vi "Process.vi"(8 "error in (no error)":errorcluster, 11 "SMO.UI":refnum<class "SMO.UI.Template.lvclass">) -> (0 "error out":errorcluster, 3 "SMO.UI out":refnum<class "SMO.UI.Template.lvclass">)   [LabVIEW 2013, in "SMO.UI.Template.lvclass"]
uses:
  SMO.UI.Template.lvclass
  SMO/Typedefs/Parent Call--Enum.ctl
  SMO.UI/SMO.UI.lvclass
  SMO/SMO.lvclass
panel:
  in  "OK":bool
  # "UI Template"
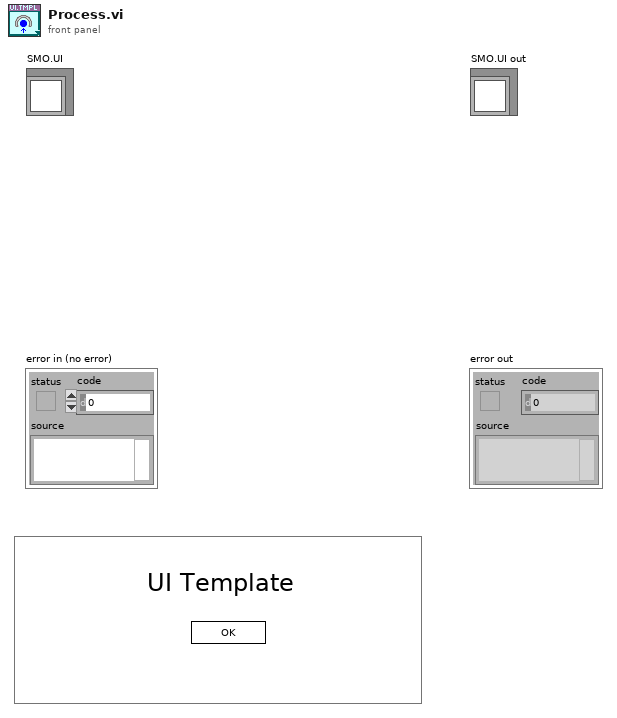
[diagram p1: front panel]
types:
  T1 = typedef "SMO.lvclass/Parent Call--Enum.ctl" = enum16{"Allows parent to run", "Does not request parent to run"}
  T2 = enum32{"invalid app kind", "Development System", "Run Time System", "Student Edition", "Embedded LabVIEW", "Evaluation", "Custom"}
  T3 = enum32{"Invalid", "Standard", "Closed", "Hidden", "Minimized", "Maximized"}
  T4 = cluster{"Core":cluster{"Current VI Reference":refnum<vi>, "Close Panel on Exit?":bool, "error":errorcluster}, "Self Ref":refnum<class "SMO.UI.Template.lvclass">}
  T5 = cluster{"Current VI Reference":refnum<vi>, "Close Panel on Exit?":bool, "error":errorcluster}
  T6 = typedef "SMO.lvclass/Protected Events.ctl" = cluster{"StopProcesses":refnum<user-event>, "AbortProcesses":refnum<user-event>}
  T7 = cluster{"Event Registration Refnum":refnum<event-registration>, "SMO.UI Public Events":refnum<event-registration>}
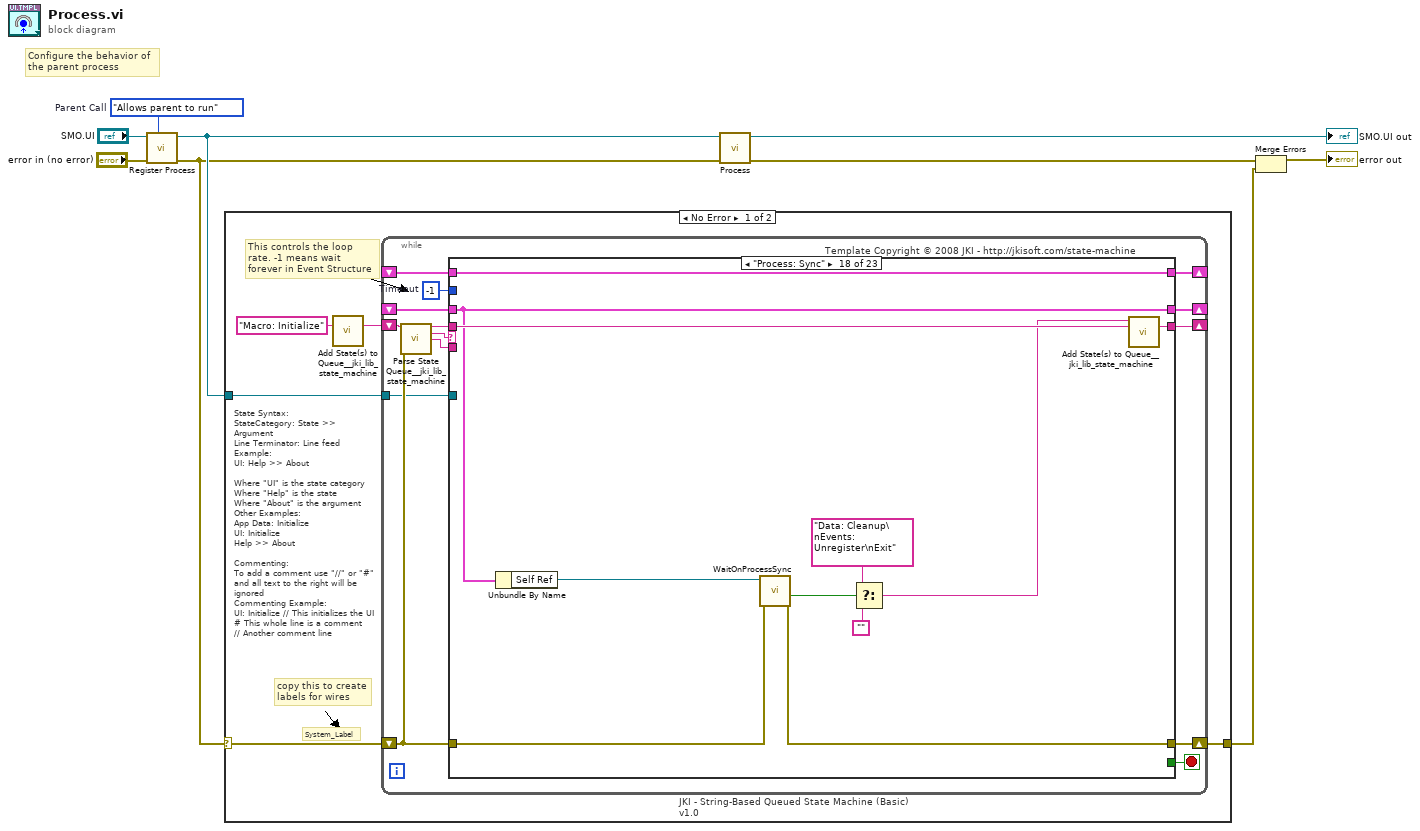
[diagram p0: block diagram]
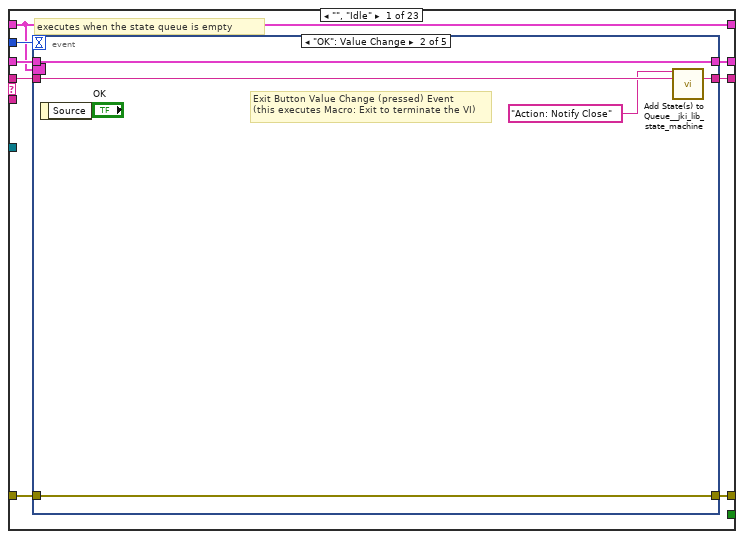
[diagram p2: hidden frame]
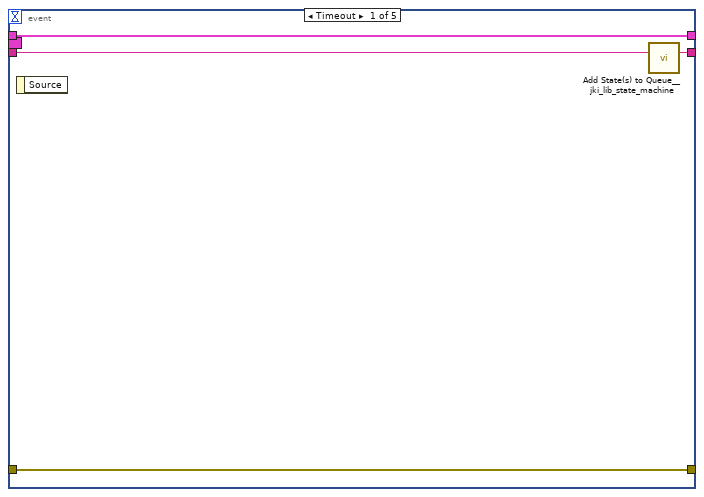
[diagram p3: hidden frame]
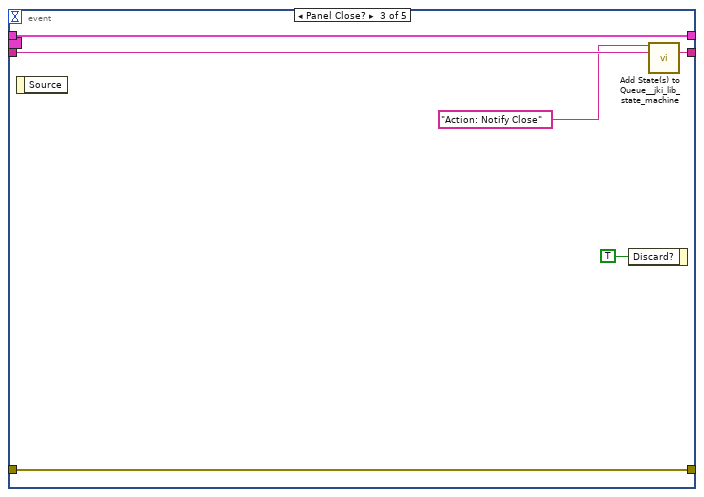
[diagram p4: hidden frame]
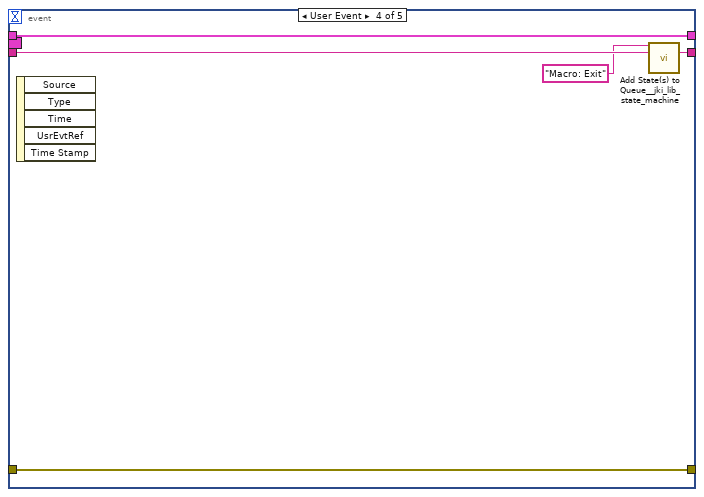
[diagram p5: hidden frame]
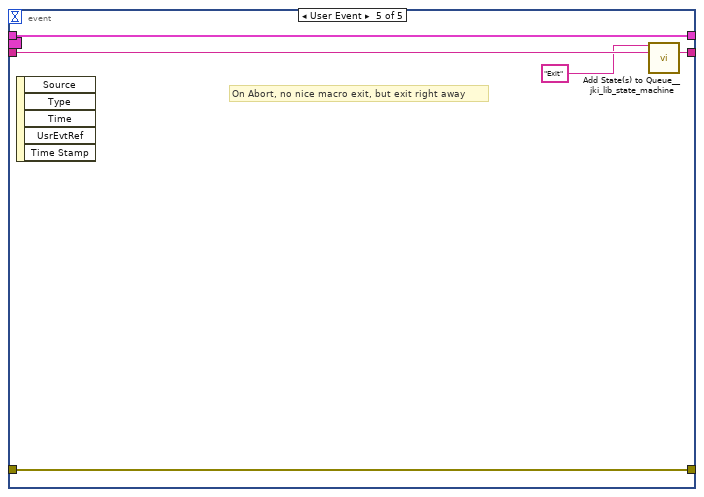
[diagram p6: hidden frame]
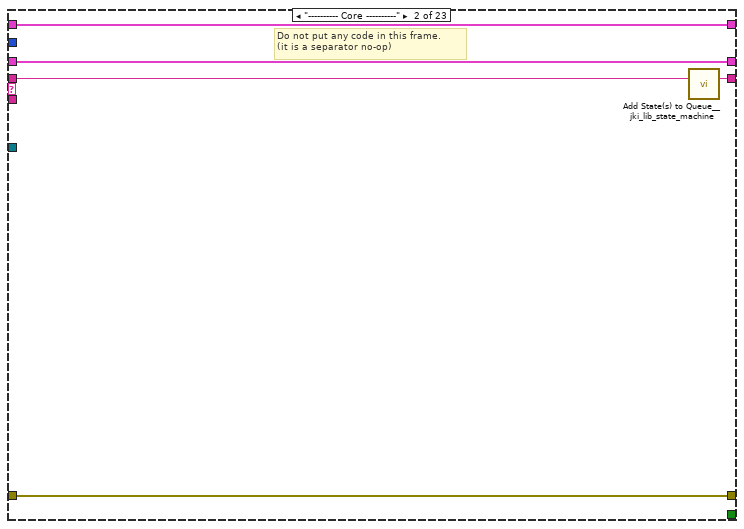
[diagram p7: hidden frame]
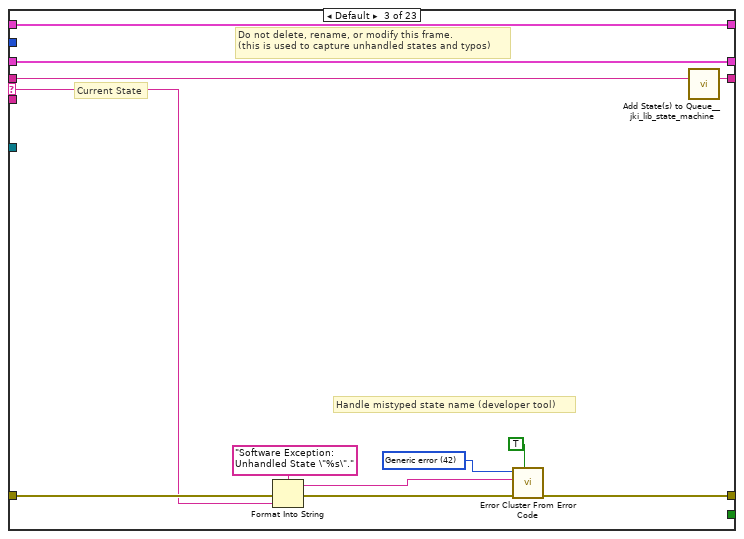
[diagram p8: hidden frame]
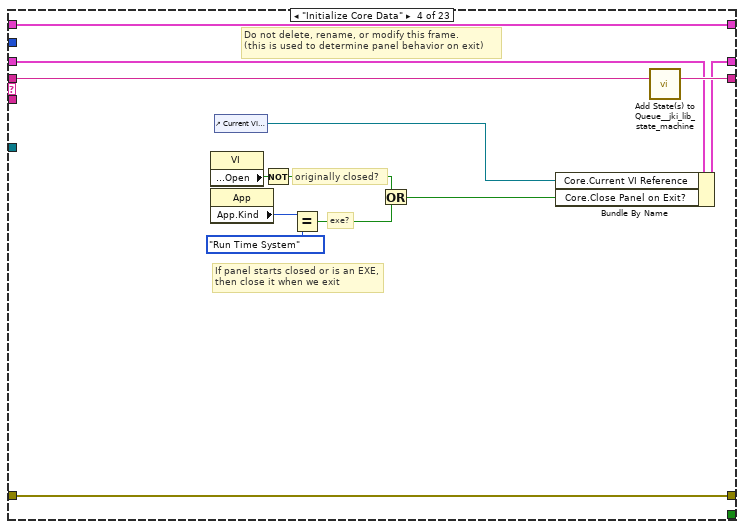
[diagram p9: hidden frame]
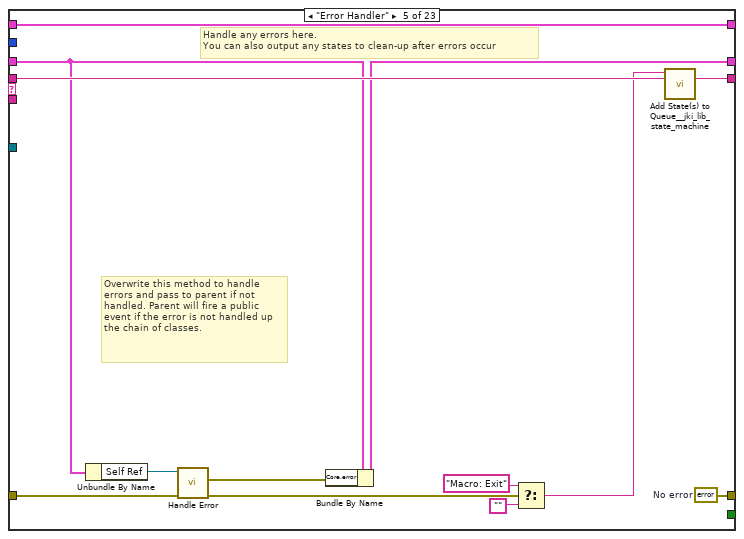
[diagram p10: hidden frame]
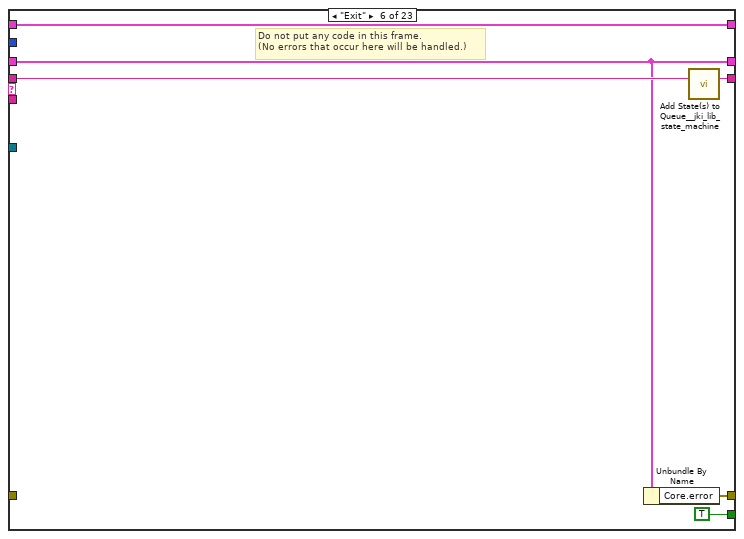
[diagram p11: hidden frame]
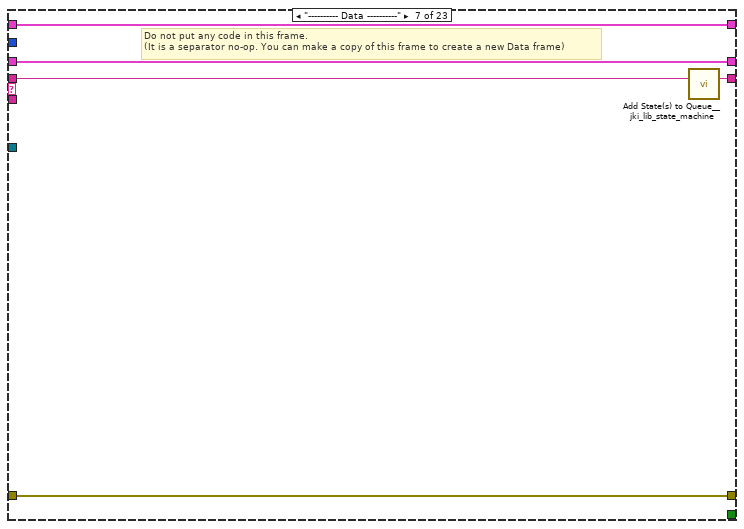
[diagram p12: hidden frame]
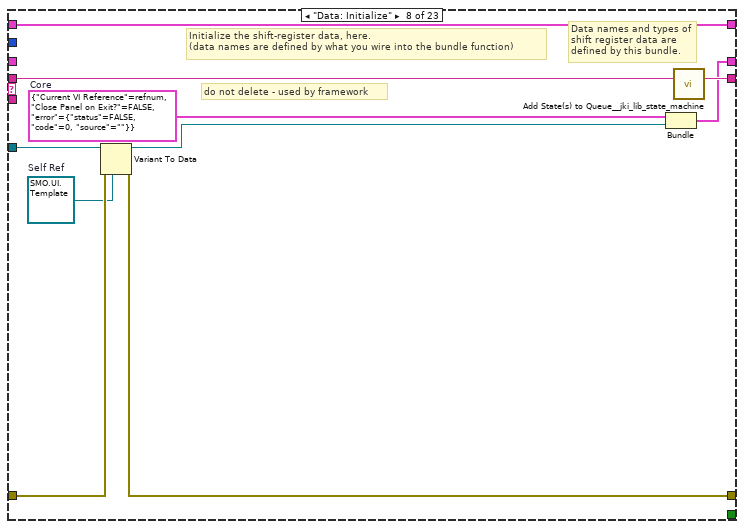
[diagram p13: hidden frame]
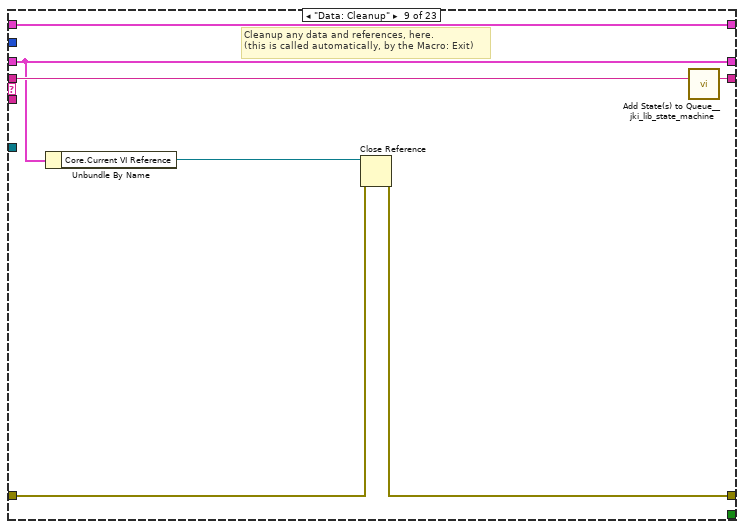
[diagram p14: hidden frame]
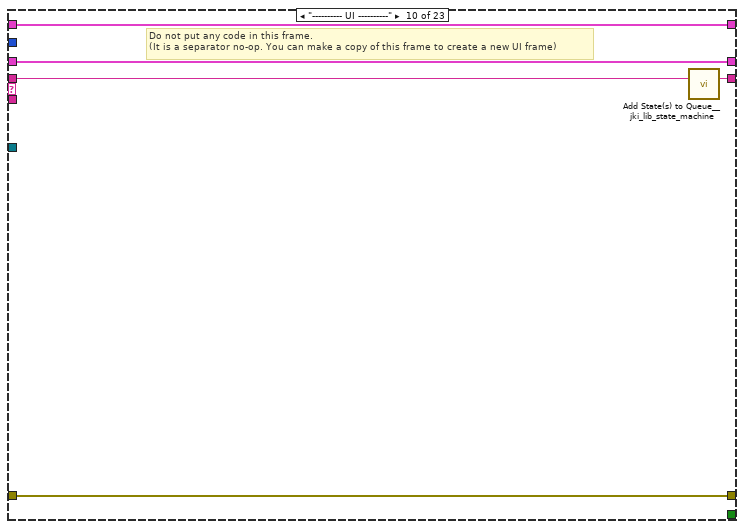
[diagram p15: hidden frame]
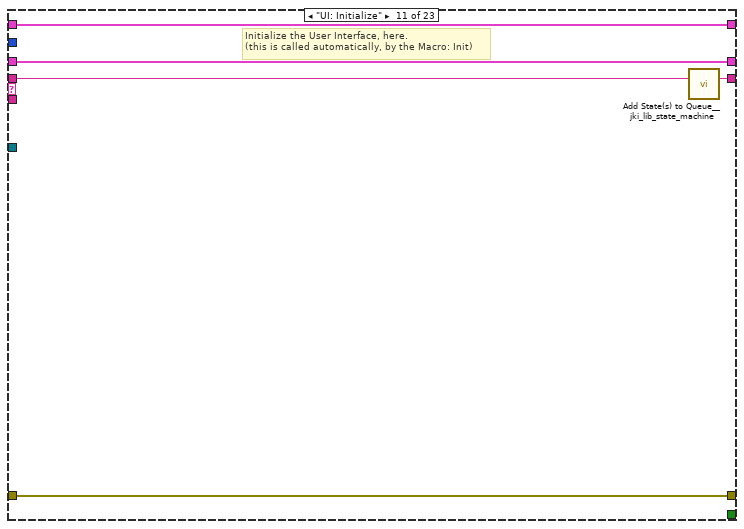
[diagram p16: hidden frame]
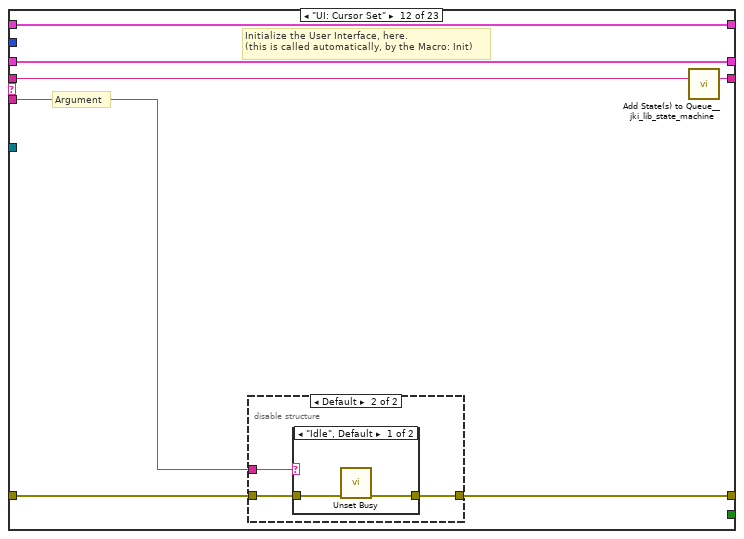
[diagram p17: hidden frame]
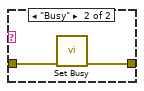
[diagram p19: hidden frame]
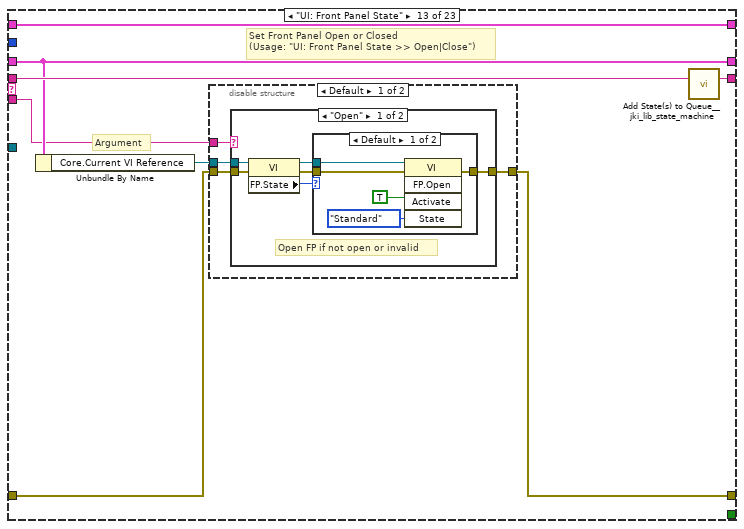
[diagram p20: hidden frame]
diagram:
  w1 = Parent_Call--Enum."Allows parent to run"  # Parent Call
  # "Configure the behavior of the parent process"
  n1 = call "Register Process.vi"("Parent Call"=w1, "error in (no error)"="error in (no error)", "SMO"="SMO.UI") -> ("error out"=w3:errorcluster, "SMO out"=w4:refnum<class "SMO.UI.Template.lvclass">)  [unwired: 7 in]
  n2 = case shown="No Error" w3 {
    selector: w3 -> [w11 w271]
    tunnel: w4 -> [w12 _]
    tunnel: [w10 w271] -> w2
    frame No Error {
      # "State Syntax:\nStateCategory: State >> Argument\nLine Terminator: Line feed\nExample:\nUI: Help >> About\n\nWhere \"UI\" is the state category\nWhere \"Help\" is the state\nWhere \"About\" is the argument\nOther Examples:\nApp Data: Initialize\nUI: Initialize\nHelp >> About\n\nCommenting:\nTo add a comment use \"//\" or \"#\" and all text to the right will be ignored\nCommenting Example:\nUI: Initialize // This initializes the UI\n# This whole line is a comment\n// Another comment line"
      # "copy this to create labels for wires"
      # "This controls the loop rate. -1 means wait forever in Event Structure"
      # "System_Label"
      n3 = call <vilib>:"Add State(s) to Queue__jki_lib_state_machine.vi"("State(s) in (\"\")"="Macro: Initialize") -> ("States Out"=w14:string)  [unwired: 14 in]
      n4 = while "JKI - String-Based Queued State Machine (Basic) v1.0" {
        shift-right: [w21] -> _
        shift-left: _ -> [w20]
        shift-right: [w24] -> w10
        shift-left: w11 -> [w18]
        shift-right: [w23] -> _
        shift-left: w14 -> [w25]
        tunnel: w12 -> [w17]
        shift-right: [w16] -> _
        shift-left: _ -> [w15]
        stop <- w22 stop-if-true
        w19 = -1  # Timeout
        # "Template Copyright © 2008 JKI - http://jkisoft.com/state-machine"
        n5 = call <vilib>:"Parse State Queue__jki_lib_state_machine.vi"("State Queue"=w25, "Error In (no error)"=w18) -> ("Remaining States"=w27:string, "Current State"=w28:string, "Arguments"=w26:string)  [unwired: 11 in]
        n6 = case shown="\"Process: Sync\"" w28 {
          selector: w28 -> [_ _ w68 _ _ _ _ _ _ _ _ _ _ _ _ _ _ _ _ _ _ _ _]
          tunnel: w27 -> [w36 w66 w72 w91 w104 w110 w115 w125 w132 w137 w142 w149 w165 w197 w206 w217 w222 w233 w238 w252 w258 w263 w270]
          tunnel: w26 -> [_ _ _ _ _ _ _ _ _ _ _ w143 w158 _ _ _ _ _ _ _ _ _ _]
          tunnel: w20 -> [w34 w63 w70 w82 w95 w106 w112 _ w127 w134 w140 w147 w163 w194 w202 w208 w219 w229 w235 w250 w256 w260 w266]
          tunnel: [w33 w64 w74 w88 w92 w105 w113 w116 w128 w135 w139 w144 w160 w195 w204 w215 w220 w230 w236 w239 w254 w261 w264] -> w24
          tunnel: w18 -> [w32 w64 w73 w88 w96 _ w113 w122 w129 w135 w139 w145 w161 w195 w204 w215 w220 w227 w236 w243 w254 w261 w265]
          tunnel: [w35 w65 w71 w90 w103 w109 w114 w124 w131 w136 w141 w148 w164 w196 w205 w216 w221 w232 w237 w251 w257 w262 w269] -> w23
          tunnel: [_ _ _ _ _ TRUE _ _ _ _ _ _ _ _ _ _ _ _ _ _ _ _ _] -> w22
          tunnel: [w31 w63 w70 w89 w94 w106 w112 w123 w127 w134 w140 w147 w163 w194 w202 w208 w219 w229 w235 w250 w256 w260 w266] -> w21
          tunnel: w19 -> [w30 _ _ _ _ _ _ _ _ _ _ _ _ _ _ _ _ _ _ _ _ _ _]
          tunnel: w17 -> [_ _ _ _ _ _ _ w121 _ _ _ _ _ _ _ _ _ _ _ _ _ _ _]
          tunnel: [w29 w62 w67 w79 w102 w107 w111 w120 w126 w133 w138 w146 w162 w193 w203 w209 w218 w231 w234 w246 w255 w259 w268] -> w16
          tunnel: w15 -> [w29 w62 w67 w79 w102 w107 w111 w120 w126 w133 w138 w146 w162 w193 w203 w209 w218 w231 w234 _ w255 w259 w268]
          frame "", "Idle" {
            # "executes when the state queue is empty"
            n7 = event shown="[1] \"OK\": Value Change" {
              selector: w29 -> [_ _ _ _ _]
              dyn-events: _ -> [_ _ _ _ _]
              timeout: w30 -> [_ _ _ _ _]
              tunnel: w36 -> [w40 w45 w51 w56 w61]
              tunnel: [w39 w44 w50 w55 w60] -> w35
              tunnel: w34 -> [w37 w42 w48 w53 w58]
              tunnel: [w38 w43 w47 w54 w59] -> w33
              tunnel: w32 -> [w38 w43 w47 w54 w59]
              tunnel: [w37 w42 w48 w53 w58] -> w31
              event Timeout {
                n8 = event-data() -> ()  [unwired: 1 in, 1 out]
                n9 = call <vilib>:"Add State(s) to Queue__jki_lib_state_machine.vi"("State(s) in (\"\")"=w40) -> ("States Out"=w39:string)  [unwired: 14 in]
              }
              event "OK": Value Change {
                # "Exit Button Value Change (pressed) Event\n(this executes Macro: Exit to terminate the VI)"
                n10 = event-data() -> ()  [unwired: 1 in, 1 out]
                n11 = call <vilib>:"Add State(s) to Queue__jki_lib_state_machine.vi"("State(s) in Front (\"\")"="Action: Notify Close", "State(s) in (\"\")"=w45) -> ("States Out"=w44:string)  [unwired: 13 in]
              }
              event Panel Close? {
                n12 = event-data() -> ()  [unwired: 1 in, 1 out]
                n13 = event-data("Discard?"=TRUE) -> ()  [unwired: 1 in, 1 out]
                n14 = call <vilib>:"Add State(s) to Queue__jki_lib_state_machine.vi"("State(s) in Front (\"\")"="Action: Notify Close" ("State(s) in Front (\"\")"), "State(s) in (\"\")"=w51) -> ("States Out"=w50:string)  [unwired: 13 in]
              }
              event User Event {
                n15 = event-data() -> ()  [unwired: 1 in, 5 out]
                n16 = call <vilib>:"Add State(s) to Queue__jki_lib_state_machine.vi"("State(s) in Front (\"\")"="Macro: Exit", "State(s) in (\"\")"=w56) -> ("States Out"=w55:string)  [unwired: 13 in]
              }
              event User Event {
                # "On Abort, no nice macro exit, but exit right away"
                n17 = event-data() -> ()  [unwired: 1 in, 5 out]
                n18 = call <vilib>:"Add State(s) to Queue__jki_lib_state_machine.vi"("State(s) in Front (\"\")"="Exit", "State(s) in (\"\")"=w61) -> ("States Out"=w60:string)  [unwired: 13 in]
              }
            }
          }
          frame "---------- Core ----------" {
            # "Do not put any code in this frame.\n(it is a separator no-op)"
            n19 = call <vilib>:"Add State(s) to Queue__jki_lib_state_machine.vi"("State(s) in (\"\")"=w66) -> ("States Out"=w65:string)  [unwired: 14 in]
          }
          frame Default {
            w77 = 42 items=["No error", "Argument error", "Memory is full", "Out of zone", "End of file", "File already open", "Generic file I/O error", "File not found", "File permission error", "Disk is full", "Duplicate path", "Too many files open", "System feature not enabled", "Resource file not found", "Cannot add resource", "Resource not found", "Image not found", "Image memory error", "Pen does not exist", "Config type invalid", "Config token not found", "Config parse error", "Config memory error", "Bad external code format", "Bad external code offset", "External code not present", "Null window", "Destroy window error", "Null menu", "Print aborted", "Bad print record", "Print driver error", "Windows error during printing", "Memory error during printing", "Print dialog error", "Generic print error", "Invalid device refnum", "Device not found", "Device parameter error", "Device unit error", "Cannot open device", "Device call aborted", "Generic error", "Cancelled by user", "Object ID too low", "Object ID too high", "Object not in heap", "Unknown heap", "Unknown object (invalid DefProc)", "Unknown object (DefProc not in table)", "Message out of range", "Invalid (null) method", "Unknown message", "Manager call not supported", "Bad address", "Network operation in progress", "Network operation timed out", "Connection is busy", "Network attribute not supported", "Network error", "Address in use", "System out of memory", "Connection aborted", "Connection refused", "Not connected", "Already connected", "Connection closed", "Initialization error (interapplication manager)", "Bad occurrence", "Wait on unbound occurrence handler", "Occurrence queue overflow", "Datalog type conflict", "Unused", "Unrecognized type (interapplication manager)", "Memory corrupt", "Failed to make temporary DLL", "Old CIN version", "Drag socket not found", "Failed to load drop-object", "Failed to register OLE object", "Failed to release OLE object", "Format specifier type mismatch", "Unknown format specifier", "Too few format specifiers", "Too many format specifiers", "Scan failed", "Newer CIN version", "Error converting to variant", "Runtime menu error", "Password tampered", "Variant attribute not found", "Incompatible variant data type", "Event data is not available", "Event Store is not present", "Occurrence is not found", "Event Queue is not created", "Event info is not available", "Refnum passed is NULL", "Error retrieving Class GUID", "Error retrieving CoClass GUID", "Error retrieving TypeLib GUID.", "Bad built application magic bytes.", "Specific driver is different from the specific driver associated with the Logical Name.", "There is no session opened to the class driver.", "Max Error", "MAX - Error with config objects", "MAX - Error loading configuration", "MAX - Group not supported"]
            # "Current State"
            # "Do not delete, rename, or modify this frame.\n(this is used to capture unhandled states and typos)"
            # "Handle mistyped state name (developer tool)"
            n20 = Format Into String(format string="Software Exception: Unhandled State \"%s\"." ("message"), error in=w73, w68) -> (resulting string=w76:string, error out=w75:errorcluster)  [unwired: 1 in]
            n21 = call <vilib>:"Error Cluster From Error Code.vi"("show call chain? (False)"=TRUE, "error in (no error)"=w75, "error message (\"\")"=w76, "error code (0)"=w77) -> ("error out"=w74:errorcluster)  [unwired: 5 in]
            n22 = call <vilib>:"Add State(s) to Queue__jki_lib_state_machine.vi"("State(s) in (\"\")"=w72) -> ("States Out"=w71:string)  [unwired: 14 in]
          }
          frame "Initialize Core Data" {
            # "Do not delete, rename, or modify this frame.\n(this is used to determine panel behavior on exit)"
            # "originally closed?"
            # "exe?"
            # "If panel starts closed or is an EXE, then close it when we exit"
            n23 = property class="VI"() -> ("Front Panel.Open"=w87:bool)  [unwired: 2 in, 2 out]
            n24 = property class="App"() -> ("App.Kind"=w86:T2)  [unwired: 2 in, 2 out]
            n25 = control-ref of="Current VI Reference"() -> (w80:refnum<vi>)
            n26 = Not(x=w87) -> (.not. x?=w84:bool)
            n27 = Equal?(x=w86, y=T2."Run Time System" ("Application:Kind")) -> (x = y?=w83:bool)
            n28 = Or(x=w84, y=w83) -> (x .or. y?=w81:bool)
            n29 = Bundle By Name(cluster=w82, "Core.Current VI Reference"=w80, "Core.Close Panel on Exit?"=w81) -> (w89:T4)
            n30 = call <vilib>:"Add State(s) to Queue__jki_lib_state_machine.vi"("State(s) in (\"\")"=w91) -> ("States Out"=w90:string)  [unwired: 14 in]
          }
          frame "Error Handler" {
            w92 = errorcluster {"status"=FALSE, "code"=0, "source"=""}  # No error
            # "Overwrite this method to handle errors and pass to parent if not handled. Parent will fire a public event if the error is not handled up the chain of classes."
            # "Handle any errors here.\nYou can also output any states to clean-up after errors occur"
            n31 = Unbundle By Name(w95) -> ("Self Ref"=w97:refnum<class "SMO.UI.Template.lvclass">)
            n32 = call-dynamic "Handle Error.vi"("error in"=w96, "SMO"=w97) -> ("handling error"=w100:errorcluster, "Unhandled error"=w101:errorcluster)  [unwired: 7 in, 1 out]
            n33 = Bundle By Name(cluster=w95, "Core.error"=w101) -> (w94:T4)
            n34 = Select(t="Macro: Exit", s=w100, f="") -> (s? t:f=w93:string)
            n35 = call <vilib>:"Add State(s) to Queue__jki_lib_state_machine.vi"("State(s) in Front (\"\")"=w93, "State(s) in (\"\")"=w104) -> ("States Out"=w103:string)  [unwired: 13 in]
          }
          frame "Exit" {
            # "Do not put any code in this frame.\n(No errors that occur here will be handled.)"
            n36 = Unbundle By Name(w106) -> ("Core.error"=w105:errorcluster)
            n37 = call <vilib>:"Add State(s) to Queue__jki_lib_state_machine.vi"("State(s) in (\"\")"=w110) -> ("States Out"=w109:string)  [unwired: 14 in]
          }
          frame "---------- Data ----------" {
            # "Do not put any code in this frame.\n(It is a separator no-op. You can make a copy of this frame to create a new Data frame)"
            n38 = call <vilib>:"Add State(s) to Queue__jki_lib_state_machine.vi"("State(s) in (\"\")"=w115) -> ("States Out"=w114:string)  [unwired: 14 in]
          }
          frame "Data: Initialize" {
            w117 = T5 {"Current VI Reference"=refnum, "Close Panel on Exit?"=FALSE, "error"={"status"=FALSE, "code"=0, "source"=""}}  # Core
            w119 = refnum<class "SMO.UI.Template.lvclass"> refnum  # Self Ref
            # "do not delete - used by framework"
            # "Data names and types of shift register data are defined by this bundle."
            # "Initialize the shift-register data, here.\n(data names are defined by what you wire into the bundle function)"
            n39 = Variant To Data(error in=w122, type=w119, Variant=w121) -> (data=w118:refnum<class "SMO.UI.Template.lvclass">, error out=w116:errorcluster)
            n40 = Bundle("Core"=w117, "Self Ref"=w118) -> (w123:T4)  [unwired: 1 in]
            n41 = call <vilib>:"Add State(s) to Queue__jki_lib_state_machine.vi"("State(s) in (\"\")"=w125) -> ("States Out"=w124:string)  [unwired: 14 in]
          }
          frame "Data: Cleanup" {
            # "Cleanup any data and references, here.\n(this is called automatically, by the Macro: Exit)"
            n42 = Unbundle By Name(w127) -> ("Core.Current VI Reference"=w130:refnum<vi>)
            n43 = Close Reference(reference=w130, error in (no error)=w129) -> (error out=w128:errorcluster)
            n44 = call <vilib>:"Add State(s) to Queue__jki_lib_state_machine.vi"("State(s) in (\"\")"=w132) -> ("States Out"=w131:string)  [unwired: 14 in]
          }
          frame "---------- UI ----------" {
            # "Do not put any code in this frame.\n(It is a separator no-op. You can make a copy of this frame to create a new UI frame)"
            n45 = call <vilib>:"Add State(s) to Queue__jki_lib_state_machine.vi"("State(s) in (\"\")"=w137) -> ("States Out"=w136:string)  [unwired: 14 in]
          }
          frame "UI: Initialize" {
            # "Initialize the User Interface, here.\n(this is called automatically, by the Macro: Init)"
            n46 = call <vilib>:"Add State(s) to Queue__jki_lib_state_machine.vi"("State(s) in (\"\")"=w142) -> ("States Out"=w141:string)  [unwired: 14 in]
          }
          frame "UI: Cursor Set" {
            # "Argument"
            # "Initialize the User Interface, here.\n(this is called automatically, by the Macro: Init)"
            n47 = disable-structure shown="Default" {
              disable-tunnel: w145 -> [w150 w153]
              disable-tunnel: [w150 w152] -> w144
              disable-tunnel: w143 -> [_ w151]
              frame condition #0 {
              }
              frame condition #1 (active) {
                n48 = case shown="\"Idle\", Default" w151 {
                  tunnel: w153 -> [w155 w157]
                  tunnel: [w154 w156] -> w152
                  frame "Idle", Default {
                    n49 = call <vilib>:"Unset Busy.vi"("error in (no error)"=w155) -> ("error out"=w154:errorcluster)  [unwired: 10 in]
                  }
                  frame "Busy" {
                    n50 = call <vilib>:"Set Busy.vi"("error in (no error)"=w157) -> ("error out"=w156:errorcluster)  [unwired: 9 in, 1 out]
                  }
                }
              }
            }
            n51 = call <vilib>:"Add State(s) to Queue__jki_lib_state_machine.vi"("State(s) in (\"\")"=w149) -> ("States Out"=w148:string)  [unwired: 14 in]
          }
          frame "UI: Front Panel State" {
            # "Argument"
            # "Set Front Panel Open or Closed\n(Usage: \"UI: Front Panel State >> Open|Close\")"
            n52 = Unbundle By Name(w163) -> ("Core.Current VI Reference"=w159:refnum<vi>)
            n53 = disable-structure shown="Default" {
              disable-tunnel: w161 -> [w169 w192]
              disable-tunnel: [w168 w192] -> w160
              disable-tunnel: w159 -> [w167 _]
              disable-tunnel: w158 -> [w166 _]
              frame condition #0 (active) {
                n54 = case shown="\"Open\"" w166 {
                  tunnel: w169 -> [w173 w186]
                  tunnel: [w175 w187] -> w168
                  tunnel: w167 -> [w174 w184]
                  frame "Open" {
                    # "Open FP if not open or invalid"
                    n55 = property class="VI"(reference=w174, error in=w173) -> (reference out=w171:refnum<vi>, error out=w172:errorcluster, "FP.State"=w170:T3)
                    n56 = case shown="Default" w170 {
                      tunnel: [w178 w181] -> w175
                      tunnel: w172 -> [w177 w181]
                      tunnel: w171 -> [w176 _]
                      frame Default {
                        n57 = invoke class="VI" method="FP.Open"(reference=w176, error in=w177, "Activate"=TRUE, "State"=T3."Standard") -> (error out=w178:errorcluster)  [unwired: 1 in, 4 out]
                      }
                      frame "Invalid", "Standard" {
                      }
                    }
                  }
                  frame "Close", Default {
                    # "Close FP is not Closed or Invalid"
                    n58 = property class="VI"(reference=w184, error in=w186) -> (reference out=w183:refnum<vi>, error out=w185:errorcluster, "FP.State"=w182:T3)
                    n59 = case shown="Default" w182 {
                      tunnel: [w188 w191] -> w187
                      tunnel: w185 -> [w188 w190]
                      tunnel: w183 -> [_ w189]
                      frame "Invalid", "Closed" {
                      }
                      frame Default {
                        n60 = invoke class="VI" method="FP.Close"(reference=w189, error in=w190) -> (error out=w191:errorcluster)  [unwired: 1 in, 2 out]
                      }
                    }
                  }
                }
              }
              frame condition #1 {
              }
            }
            n61 = call <vilib>:"Add State(s) to Queue__jki_lib_state_machine.vi"("State(s) in (\"\")"=w165) -> ("States Out"=w164:string)  [unwired: 14 in]
          }
          frame "---------- Macro ----------" {
            # "Do not put any code in this frame.\n(It is a separator no-op. You can make a copy of this frame to create a new Macro frame)"
            n62 = call <vilib>:"Add State(s) to Queue__jki_lib_state_machine.vi"("State(s) in (\"\")"=w197) -> ("States Out"=w196:string)  [unwired: 14 in]
          }
          frame "Macro: Initialize" {
            w200 = "UI: Initialize\n//UI: Front Panel State >> Open"  # UI: Initialize //UI: Front Panel State >> Open
            # "Initialization Macro\n(This is called once, when the VI starts)"
            n63 = call <vilib>:"Add State(s) to Queue__jki_lib_state_machine.vi"("State(s) in Front (\"\")"="Data: Initialize\nInitialize Core Data\nEvents: Register", "State(s) in (\"\")"="Process: Sync", "State(s) at Back (\"\")"=w200) -> ("States Out"=w199:string)  [unwired: 12 in]
            n64 = call <vilib>:"Add State(s) to Queue__jki_lib_state_machine.vi"("State(s) in Front (\"\")"=w199, "State(s) in (\"\")"=w206) -> ("States Out"=w205:string)  [unwired: 13 in]
          }
          frame "Macro: Exit" {
            # "Exit Macro\n(This is called once, when the VI exits)"
            n65 = Unbundle By Name(w208) -> ("Core.Close Panel on Exit?"=w214:bool)
            n66 = Select(t="//UI: Front Panel State >> Close", s=w214, f="") -> (s? t:f=w211:string)
            n67 = call <vilib>:"Add State(s) to Queue__jki_lib_state_machine.vi"("State(s) in (\"\")"=w211, "State(s) at Back (\"\")"="Data: Cleanup\nEvents: Unregister\nProcess: Sync\nExit") -> ("States Out"=w210:string)  [unwired: 13 in]
            n68 = call <vilib>:"Add State(s) to Queue__jki_lib_state_machine.vi"("State(s) in Front (\"\")"=w210, "State(s) in (\"\")"=w217) -> ("States Out"=w216:string)  [unwired: 13 in]
          }
          frame "---------- Process ----------" {
            # "Template Separator\n(You can make a copy of, or modify, this frame)"
            n69 = call <vilib>:"Add State(s) to Queue__jki_lib_state_machine.vi"("State(s) in (\"\")"=w222) -> ("States Out"=w221:string)  [unwired: 14 in]
          }
          frame "Process: Sync" {
            n70 = Unbundle By Name(w229) -> ("Self Ref"=w228:refnum<class "SMO.UI.Template.lvclass">)
            n71 = call "WaitOnProcessSync.vi"("error in (no error)"=w227, "SMO"=w228) -> ("error out"=w230:errorcluster, "Don't run?"=w226:bool)  [unwired: 7 in, 1 out]
            n72 = Select(t="Data: Cleanup\nEvents: Unregister\nExit", s=w226, f="") -> (s? t:f=w223:string)
            n73 = call <vilib>:"Add State(s) to Queue__jki_lib_state_machine.vi"("State(s) in Front (\"\")"=w223, "State(s) in (\"\")"=w233) -> ("States Out"=w232:string)  [unwired: 13 in]
          }
          frame "---------- Events ----------" {
            # "Template Separator\n(You can make a copy of, or modify, this frame)"
            n74 = call <vilib>:"Add State(s) to Queue__jki_lib_state_machine.vi"("State(s) in (\"\")"=w238) -> ("States Out"=w237:string)  [unwired: 14 in]
          }
          frame "Events: Register" {
            # "Base Class Protected Events"
            # "Your code here.\n(You can make a copy of, or modify, this frame)"
            n75 = Unbundle By Name(w250) -> ("Self Ref"=w248:refnum<class "SMO.UI.Template.lvclass">)
            n76 = call "GetProtectedEvents.vi"("SMO"=w248) -> ("error out"=w240:errorcluster, "SMO Protected Events"=w249:T6, "SMO out"=w245:refnum<class "SMO.UI.Template.lvclass">)  [unwired: 8 in]
            n77 = call "SMO.UI.GetPublicEventsRegistration.vi"("SMO.UI"=w245) -> ("error out"=w241:errorcluster, "SMO.UI Public Events"=w244:refnum<event-registration>)  [unwired: 8 in, 1 out]
            n78 = register-events(w249) -> (reference out=w247:refnum<event-registration>, error out=w242:errorcluster)  [unwired: 2 in]
            n79 = Merge Errors(w242, w241, w240, w243) -> (w239:errorcluster)
            n80 = Bundle("Event Registration Refnum"=w247, "SMO.UI Public Events"=w244) -> (w246:T7)  [unwired: 1 in]
            n81 = call <vilib>:"Add State(s) to Queue__jki_lib_state_machine.vi"("State(s) in (\"\")"=w252) -> ("States Out"=w251:string)  [unwired: 14 in]
          }
          frame "Events: Unregister" {
            n82 = Unregister For Events(event registration refnum=w255, error in=w254) -> (error out=w253:errorcluster)
            n83 = call <vilib>:"Clear Errors.vi"("error in (no error)"=w253) -> ()  [unwired: 6 in, 1 out]
            n84 = call <vilib>:"Add State(s) to Queue__jki_lib_state_machine.vi"("State(s) in (\"\")"=w258) -> ("States Out"=w257:string)  [unwired: 14 in]
          }
          frame "---------Action---------" {
            # "Action Separator\n(You can make a copy of, or modify, this frame)"
            n85 = call <vilib>:"Add State(s) to Queue__jki_lib_state_machine.vi"("State(s) in (\"\")"=w263) -> ("States Out"=w262:string)  [unwired: 14 in]
          }
          frame "Action: Notify Close" {
            # "Notify that the UI has been closed"
            n86 = Unbundle By Name(w266) -> ("Self Ref"=w267:refnum<class "SMO.UI.Template.lvclass">)
            n87 = call "Hide.vi"("error in (no error)"=w265, "SMO.UI"=w267) -> ("error out"=w264:errorcluster)  [unwired: 8 in, 1 out]
            n88 = call <vilib>:"Add State(s) to Queue__jki_lib_state_machine.vi"("State(s) in (\"\")"=w270) -> ("States Out"=w269:string)  [unwired: 14 in]
          }
        }
      }
    }
    frame Error {
    }
  }
  n89 = call-parent "Process.vi"("error in (no error)"=w3, "SMO.UI"=w4) -> ("error out"=w9:errorcluster, "SMO.UI out"=→"SMO.UI out":refnum<class "SMO.UI.Template.lvclass">)  [unwired: 8 in]
  n90 = Merge Errors(w9, w2) -> (→"error out":errorcluster)
